vi "Set Disable Refresh Modules.vi"(8 "error in":errorcluster, 10 "disable refresh modules":bool, 11 "scan engine custom device ref in":T1 format="%.0x") -> (0 "error out":errorcluster, 3 "scan engine custom device ref out":T1 format="%.0x")   [LabVIEW 2020, in "Scan Engine Scripting.lvlib"]
doc: "Writes <B>disable refresh modules</B> into the provided Scan Engine custom device reference."
uses:
  Scan Engine Scripting.lvlib
  <vilib>/NI VeriStand/Custom Device API/Custom Device Item Ref.ctl
  Shared/Globals/Property Strings.vi
  <vilib>/NI VeriStand/Custom Device API/Set Item Property (Boolean).vi
  Shared/SEECD Shared.lvlib
  <vilib>/NI VeriStand/Custom Device API/Custom Device API.lvlib
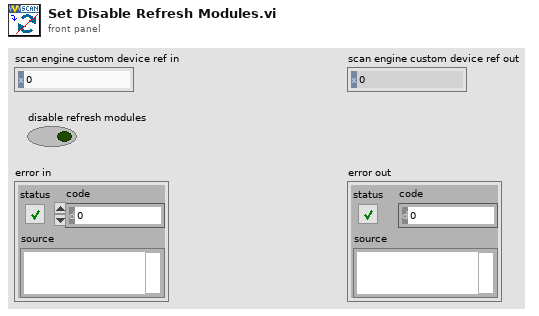
[diagram p1: front panel]
types:
  T1 = typedef "Custom Device API.lvlib/Custom Device Item Ref.ctl" = u64
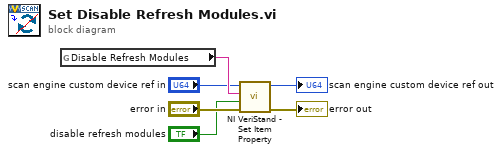
[diagram p0: block diagram]
diagram:
  n1 = global read "Property Strings.vi" "Disable Refresh Modules"() -> (w6:string)
  n2 = call-poly <vilib>:"NI VeriStand - Set Item Property.vi"("error in (no error)"="error in", "Value"="disable refresh modules", "Property Name"=w6, "Item Ref in"="scan engine custom device ref in") -> ("error out"=→"error out":errorcluster, "Item Ref out"=→"scan engine custom device ref out":T1)  [unwired: 5 in, 1 out]
